vi "UART 8N1 Credentials Response.vi"(6 "Response Timeout (ms)":i32 min=0, 7 "Enum":T1, 8 "Error In":errorcluster, 11 "FPGA VI Reference In":refnum<k20>) -> (0 "Error Out":errorcluster, 1 "Initial PAC (Hex)":string, 2 "Device ID (Hex)":string, 3 "FPGA VI Reference Out":refnum<k20>, 4 "Init Resp":string, 5 "Get Cred OK":bool, 9 "Elements Remaining":u32)   [LabVIEW 2018]
uses:
  Resources_Test/UART/ControlTestSlot.ctl
  <vilib>/Utility/error.llb/Error Cluster From Error Code.vi
  <vilib>/rvi/errors/niLvFpgaAdjustHostInterfaceError.vi
  <vilib>/rvi/interface/nirviMethod/nirviMethod.xnode
  Program Files (x86)/National Instruments/LabVIEW 2018/instr.lib/niVST/FPGA/Templates/FPGA Bitfiles/niVSTFPGA_UART.lvbitx
  <vilib>/FPGAPlugInAG/PXIe-5840/niLvFpga_ReadFifo_PXIe-5840.vi
  <vilib>/rvi/errors/niLvFpgaMergeErrorWithErrorCode.vi
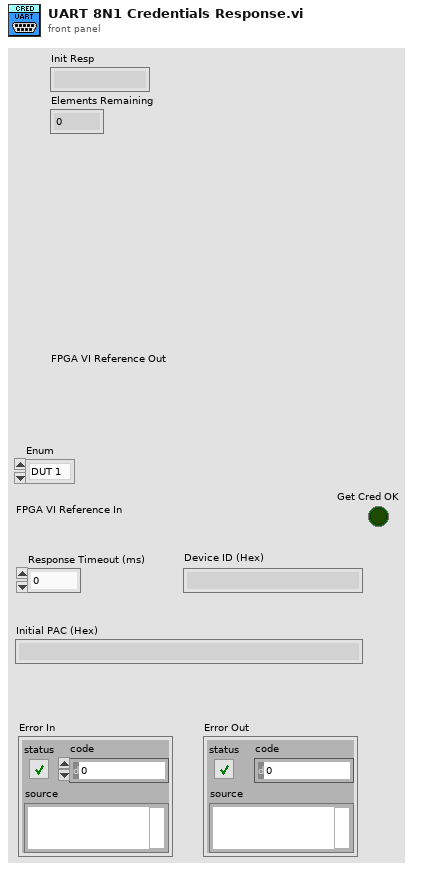
[diagram p1: front panel]
types:
  T1 = typedef "ControlTestSlot.ctl" = enum16{"DUT 1", "DUT 2"}
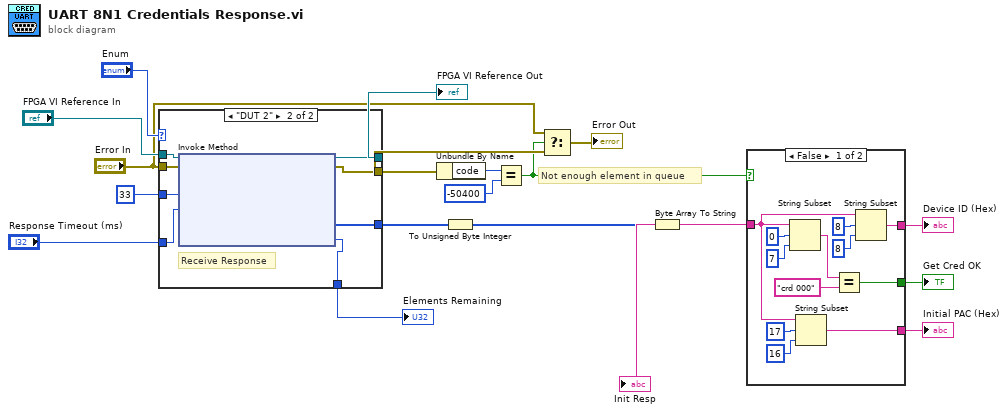
[diagram p0: block diagram]
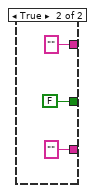
[diagram p2: hidden frame]
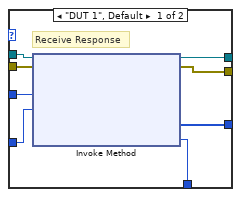
[diagram p3: hidden frame]
diagram:
  # "Not enough element in queue"
  n1 = case shown="\"DUT 2\"" "Enum" {
    tunnel: [w24 w34] -> w6
    tunnel: "Error In" -> [w23 w33]
    tunnel: "FPGA VI Reference In" -> [w26 w32]
    tunnel: u32 33 ("Response Timeout (ms)") -> [w22 w31]
    tunnel: "Response Timeout (ms)" -> [w21 w30]
    tunnel: [w25 w29] -> w10
    tunnel: [w20 w28] -> w9
    tunnel: [w19 w27] -> w1
    frame "DUT 1", Default {
      # "Receive Response"
      n2 = xnode "Invoke Method"("FPGA VI Reference In"=w26, "error in"=w23, "Number of Elements"=w22, "Timeout (ms)"=w21) -> ("FPGA VI Reference Out"=w25:refnum<k20>, "error out"=w20:errorcluster, "Data"=w24:u32[], "Elements Remaining"=w19:u32)
    }
    frame "DUT 2" {
      # "Receive Response"
      n3 = xnode "Invoke Method"("FPGA VI Reference In"=w32, "error in"=w33, "Number of Elements"=w31, "Timeout (ms)"=w30) -> ("FPGA VI Reference Out"=w29:refnum<k20>, "error out"=w28:errorcluster, "Data"=w34:u32[], "Elements Remaining"=w27:u32)
    }
  }
  "FPGA VI Reference Out" <- w10
  "Elements Remaining" <- w1
  n4 = Unbundle By Name(w9) -> ("code"=w15:i32)
  n5 = To Unsigned Byte Integer(number=w6) -> (unsigned 8bit integer=w17:u8[])
  n6 = Equal?(x=w15, y=-50400) -> (x = y?=w2:bool)
  n7 = Select(t="Error In", s=w2, f=w9) -> (s? t:f=→"Error Out":errorcluster)
  n8 = Byte Array To String(unsigned byte array=w17) -> (string=w18:string)
  "Init Resp" <- w18
  n9 = case shown="False" w2 {
    tunnel: w18 -> [w38 _]
    tunnel: [w35 FALSE] -> w5
    tunnel: [w37 "" ("string")] -> w4
    tunnel: [w36 "" ("string")] -> w3
    frame False {
      n10 = String Subset(string=w38, offset (0)=0, length (rest)=7 ("length (rest)")) -> (substring=w43:string)
      n11 = String Subset(string=w38, offset (0)=17, length (rest)=16 ("length (rest)")) -> (substring=w36:string)
      n12 = Equal?(x=w43, y="crd 000") -> (x = y?=w35:bool)
      n13 = String Subset(string=w38, offset (0)=8, length (rest)=8 ("length (rest)")) -> (substring=w37:string)
    }
    frame True {
    }
  }
  "Get Cred OK" <- w5
  "Device ID (Hex)" <- w4
  "Initial PAC (Hex)" <- w3
